vi "PDF_Interface_PDF Protokoll EPA1065_305 ARN.vi"(7 "ResultPictures":T1, 8 "error in (no error)":errorcluster caption="Fehler (Eingang, kein Fehler)", 9 "SVGraph Referenz":refnum<vi>, 10 "Save PDF File Path":path, 11 "Tabelle":string[][](table)) -> (0 "error out":errorcluster caption="Fehler (Ausgang)")   [LabVIEW 2020, in "EPA 1065.lvlib" / "ARN Test 1065-305.lvlib"]
uses:
  ARN Test 1065-305.lvlib
  T90 1065-308/Ergebnis.ctl
  PDF_Interface/PDF Interface Helper/PDFResultPictures.ctl
  Sprachverwaltung/FGV Aktion Tabelle zerlegen.ctl
  Seiten/FT-IR/FGV FT-IR Gasliste Aktionen.ctl
  Seiten/FT-IR/FGV FT-IR Aktionen.ctl
  Aktion FGV ARN Daten.ctl
  Seiten/System Einstellungen V2/Aktioen FGV System Konstanten.ctl
  PDF_Interface/PDF Protokoll Standard Kopf Optionen.ctl
  Visualisierungs Elemente/Auswahlfeld.ctl
  PDF_Interface/PDF Protokoll Standard Kopf Gasflasche Auswahl.ctl
  Aktion FGV Protokoll.ctl
  PDF_Interface/PDF Interface Helper/PDFGraph.ctl
  <vilib>/Simplicity AI/SAI_PDF_API/Classes/Context/Controls/SAI_PDF_Text Align.ctl
  PDF_Interface/PDF Interface Helper/PDFCommentPosition.ctl
  PDF_Interface/PDF Interface Helper/PDFPageBreak.ctl
  <vilib>/Simplicity AI/SAI_PDF_API/Classes/Context/Controls/SAI_PDF_PDF Details.ctl
  PDF_Interface/PDF Interface Helper/PDFContentType.ctl
  PDF_Interface/PDF Interface Helper/PDFTableContentType.ctl
  PDF_Interface/PDF Interface Helper/PDFResults.ctl
  PDF_Interface/PDF Interface Helper/PDFTablePictures.ctl
  PDF_Interface/PDF Interface Helper/PDFBemerkung.ctl
  <vilib>/Simplicity AI/SAI_PDF_API/Classes/Context/Controls/SAI_PDF_Font.ctl
  <vilib>/Simplicity AI/SAI_PDF_API/Classes/Context/Controls/SAI_PDF_Font Encoding.ctl
  Allgemein/allgemeine Sub-VIs.lvlib
  Seiten/FT-IR/FT-IR.lvlib
  Seiten/System Einstellungen V2/System Einstellungen V2.lvlib
  Sprachverwaltung/Sprachverwaltung.lvlib
  PDF_Interface/PDF Interface.lvlib
  PDF_Interface/PDF Interface Helper/PDF Interface Helper.lvlib
  <vilib>/Simplicity AI/SAI_PDF_API/Classes/Context/Context.lvclass
  Linearisierung V2/Protokoll/Protokoll.lvlib
  T90 1065-308/T90 Test 1065-308.lvlib
panel:
  out "Versa Serial number:":string caption="Serial number:"
  out "Anlage:":string caption="Measuring Device:"
  out "Einheit Noise 2":string
  out "Einheit Wiederh. 2":string
  out "Einheit Genauigkeit 2":string
  out "Einheit Noise":string
  out "Einheit Wiederh.":string
  out "Ergebnis 3":T2
  out "Ergebnis 2":T2
  out "Ergebnis 1":T2
  out "Rauschen":string
  out "Rauschen Grenze":string caption="Noise:"
  out "Wiederholgenauigkeit":string
  out "Genauigkeit":string
  out "Wiederholgenauigkeit Grenze":string caption="Repeatability:"
  out "Genauigkeit Grenze":string caption="Accuracy:"
  out "Einheit Genauigkeit":string
  out "Tabelle":string[][](table)
  out "Methode (Recipe):":string caption="Method (Recipe):"
  out "Date & Time:":string
  out "Accuracy:":string
  out "Gas Bottle Nr.:":string
  out "T90 Result":waveform(dbl)(graph) caption="T90"
  out "Ergebnis:":string caption="Result:"
  out "Konzentration:":string caption="Setpoint:"
  out "Komponente:":string caption="Component:"
  out "Bearbeiter:":string caption="Operator:"
  out "Serial number:":string
  out "Messgerät:":string caption="Analyzer:"
  # "ANR EPA § 1065.305"
  # "Limits"
  # "Results"
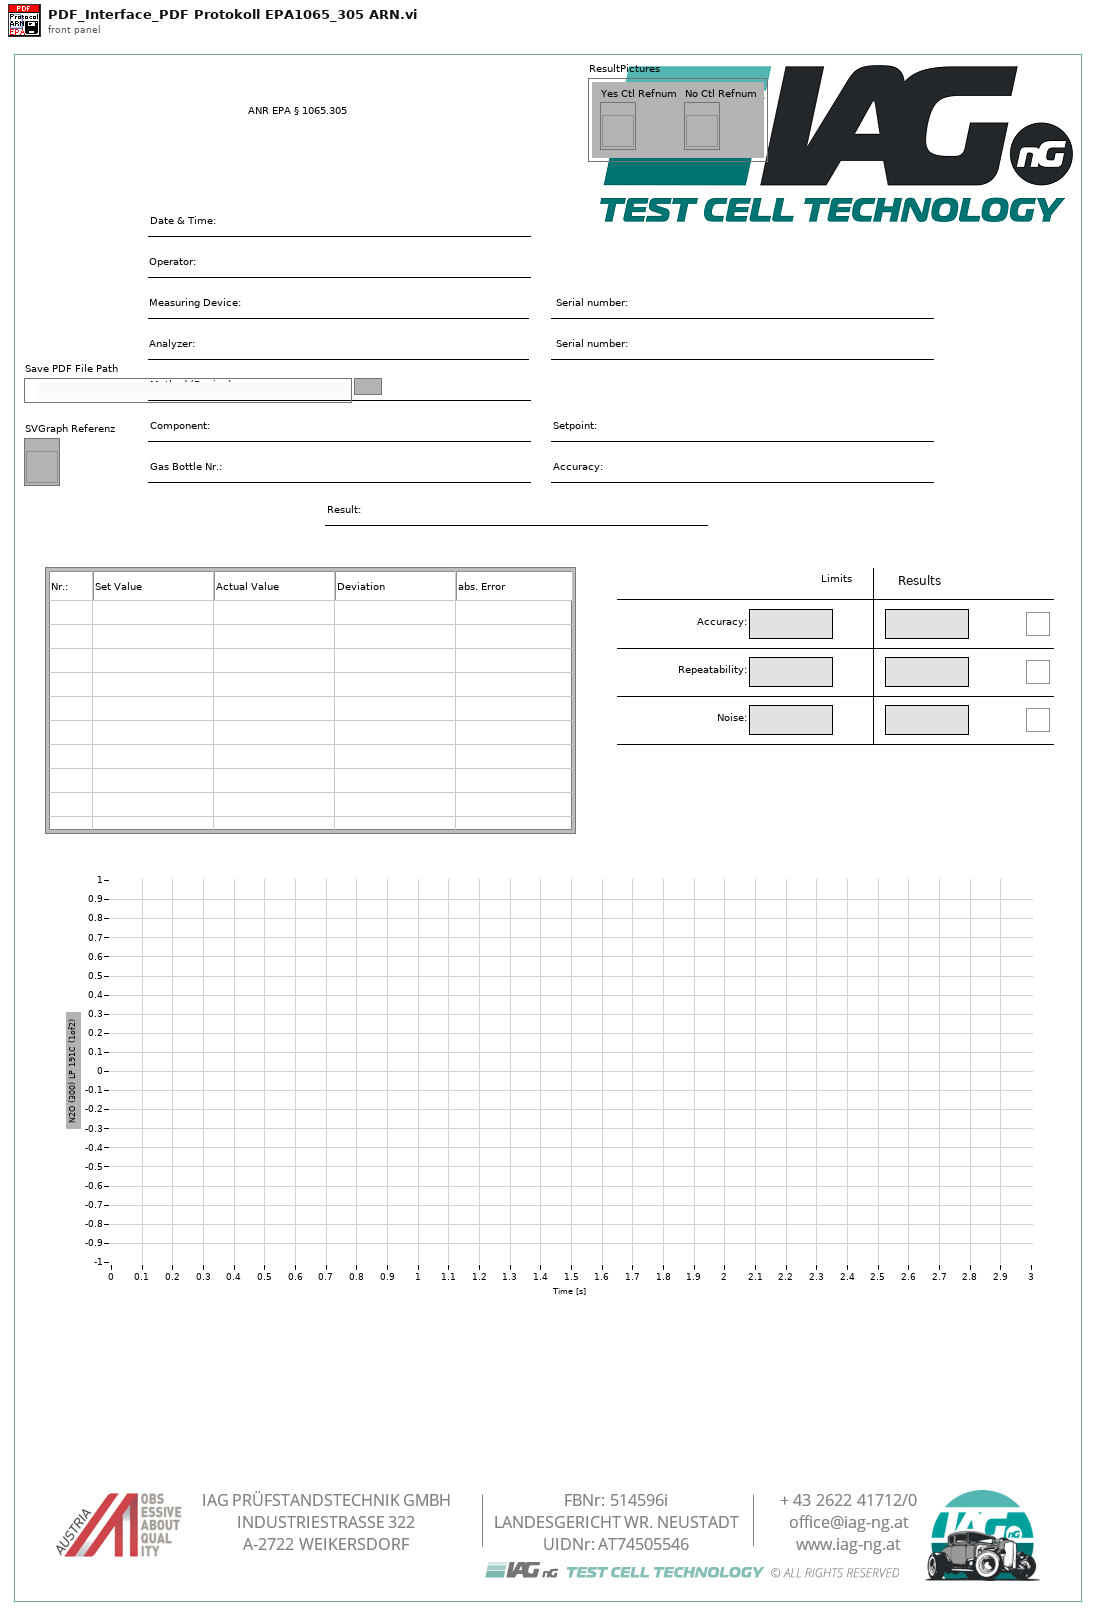
[diagram p1: front panel]
types:
  T1 = typedef "PDF Interface.lvlib/PDF Interface Helper.lvlib/PDFResultPictures.ctl" = cluster{"Yes Ctl Refnum":refnum<vi>, "No Ctl Refnum":refnum<vi>}
  T2 = typedef "EPA 1065.lvlib/T90 Test 1065-308.lvlib/Ergebnis.ctl" = bool
  T3 = typedef "Sprachverwaltung.lvlib/FGV Aktion Tabelle zerlegen.ctl" = enum16{"laden", "vereinzeln", "speichern"}
  T4 = typedef "PDF Interface.lvlib/PDF Protokoll Standard Kopf Gasflasche Auswahl.ctl" = cluster{"Gasflaschen Name":string, "Gasflaschen Nummer":string, "Gasnummer Index":i32}
  T5 = typedef "Auswahlfeld.ctl" = u16
  T6 = typedef "PDF Interface.lvlib/PDF Protokoll Standard Kopf Optionen.ctl" = cluster{"Analysator":bool, "FT-IR Rezept":bool, "Gasteiler":bool, "Gas Komponente":bool, "Gas Flasche":bool, "LIN Protokoll":bool, "Operator":bool}
  T7 = typedef "System Einstellungen V2.lvlib/Aktioen FGV System Konstanten.ctl" = enum16{"lesen", "laden", "speichern", "Sprache"}
  T8 = typedef "EPA 1065.lvlib/ARN Test 1065-305.lvlib/Aktion FGV ARN Daten.ctl" = enum16{"Lesen", "laden", "speichern", "ARN Daten", "Rohdaten", "Rohdaten löschen", "Zeitstempel", "SNR Ergebnis"}
  T9 = typedef "FT-IR.lvlib/FGV FT-IR Aktionen.ctl" = enum16{"lesen", "NOG setzen", "NOS setzen", "Initialisieren", "speichern", "ALLES setzen", "FT-IR Spektrum loggen", "Komm Stoppen", "Spektrum LogKonfig"}
  T10 = typedef "FT-IR.lvlib/FGV FT-IR Gasliste Aktionen.ctl" = enum16{"lesen", "Gasliste FT-IR", "Gasliste ausgelesen", "laden", "speichern", "löschen"}
  T11 = typedef "EPA 1065.lvlib/ARN Test 1065-305.lvlib/Aktion FGV Protokoll.ctl" = enum16{"lesen", "schreiben", "Graph"}
  T12 = typedef "PDF Interface.lvlib/PDF Interface Helper.lvlib/PDFBemerkung.ctl" = cluster{"Bemerkung Text":string, "Align (Left)":T13, "Add Line Feeds (F:No)":bool, "Font":T14}
  T13 = typedef "SAI_PDF_Toolkit.lvlib/Context.lvclass/SAI_PDF_Text Align.ctl" = i32
  T14 = typedef "SAI_PDF_Toolkit.lvlib/Context.lvclass/SAI_PDF_Font.ctl" = cluster{"Font":string, "Size":i32, "Colour":u32, "Bold":bool, "Italic":bool, "Underline":bool, "Strikethrough":bool, "Font Encoding":T15}
  T15 = typedef "SAI_PDF_Toolkit.lvlib/Context.lvclass/SAI_PDF_Font Encoding.ctl" = enum16{"Cp1252, WinANSI", "IdentityH", "IdentityV", "Cp1250", "Cp1257", "MacRoman"}
  T16 = typedef "PDF Interface.lvlib/PDF Interface Helper.lvlib/PDFContentType.ctl" = cluster{"Titel":string, "Header Table":string[][], "Table Array":T17[], "Bemerkungen":T12[]}
  T17 = typedef "PDF Interface.lvlib/PDF Interface Helper.lvlib/PDFTableContentType.ctl" = cluster{"TableHeader":string[], "Table":string[][], "Relative Column Widths (%)":sgl[], "Results":T18, "PositionBemerkung":T19, "PageBreak":T20, "TablePictures":T21, "Horizontal Align":i32}
  T18 = typedef "PDF Interface.lvlib/PDF Interface Helper.lvlib/PDFResults.ctl" = cluster{"Results":cluster{"Result Text":string, "Result":bool}[], "ResultPictures":T1, "use Pictures":bool, "Image Scale (%)":sgl, "Autoscale? (T)":bool, "Horizontal Align":i32, "Position":i32}
  T19 = typedef "PDF Interface.lvlib/PDF Interface Helper.lvlib/PDFCommentPosition.ctl" = enum16{"before", "after"}
  T20 = typedef "PDF Interface.lvlib/PDF Interface Helper.lvlib/PDFPageBreak.ctl" = enum16{"none", "before", "after", "after comment"}
  T21 = typedef "PDF Interface.lvlib/PDF Interface Helper.lvlib/PDFTablePictures.ctl" = cluster{"Ctl Refnum In":refnum<vi>[], "RowOrColumn":enum16{"Row", "Column"}, "IndexToInsert":u16, "Image Scale (%)":sgl[], "Autoscale? (T)":bool[], "Horizontal Align":i32}
  T22 = typedef "SAI_PDF_Toolkit.lvlib/Context.lvclass/SAI_PDF_PDF Details.ctl" = cluster{"Title":string, "Subject":string, "Keywords":string, "Author":string, "Creator":string}
  T23 = cluster{"Header Footer Text Cluster":cluster{"Header Text":string, "Footer Text":string, "Time":string, "Page Number":string}, "PDF Details":T22}
  T24 = typedef "EPA 1065.lvlib/ARN Test 1065-305.lvlib/Allgemeine Einstellungen.ctl" = cluster{"Bearbeiter:":string, "Analysator":T25, "Komponente:":u16, "Gasflaschen Nr.:":string, "Accuracy":dbl, "Sollwert":dbl, "Modus":T26, "Pfad:":path, "Textname:":string, "CG Aufschaltzeit:":dbl, "Einheit":string, "N2 Aufschaltzeit:":dbl, "Gasflasche":T27, "Konfig Gasflasche":T28}
  T25 = typedef "System Einstellungen V2.lvlib/Analysatoren.ctl" = string
  T26 = typedef "EPA 1065.lvlib/T90 Test 1065-308.lvlib/Modus.ctl" = u16
  T27 = typedef "System Einstellungen V2.lvlib/Gasflasche Auswahl.ctl" = u16
  T28 = typedef "System Einstellungen V2.lvlib/Konfig Gasflasche.ctl" = bool
  T29 = cluster{"Modell":string, "ProjektNummer":string, "Software Version":string, "Seriennummer":string}
  T30 = typedef "String - Ausgabefeld.ctl" = string
  T31 = cluster{"Header Size":i32, "Column Ratio left":sgl[]}
  T32 = typedef "PDF Interface.lvlib/PDF Interface Helper.lvlib/PDFGraph.ctl" = cluster{"GraphCtl Refnum":refnum<vi>, "Wrap Text (F:No)":bool, "Hide Grid (F:No)":bool, "Scale (100%)":sgl, "Align (Left)":T13, "PositionBemerkung":T19, "PageBreak":T20}
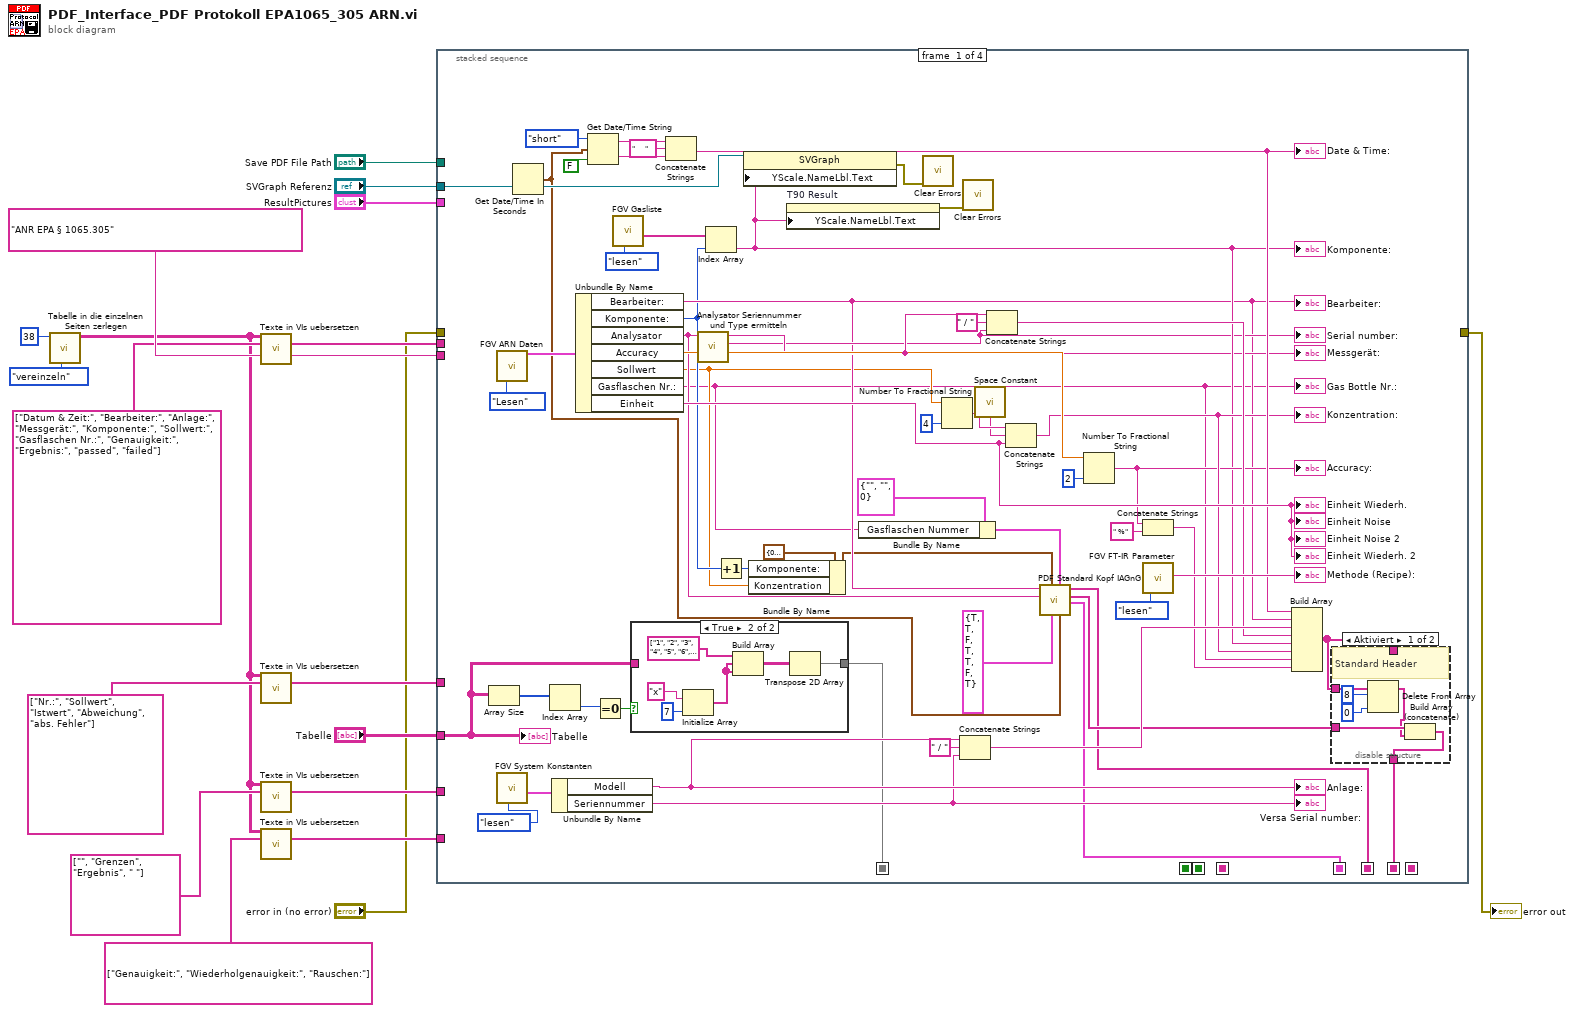
[diagram p0: block diagram]
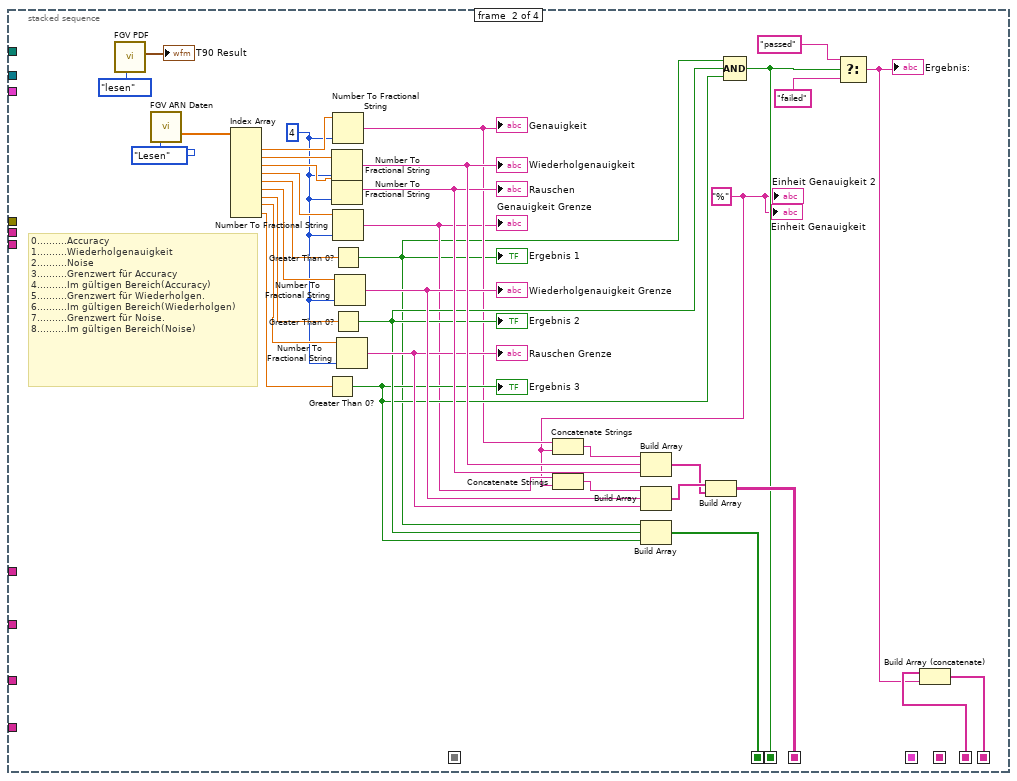
[diagram p4: hidden frame]
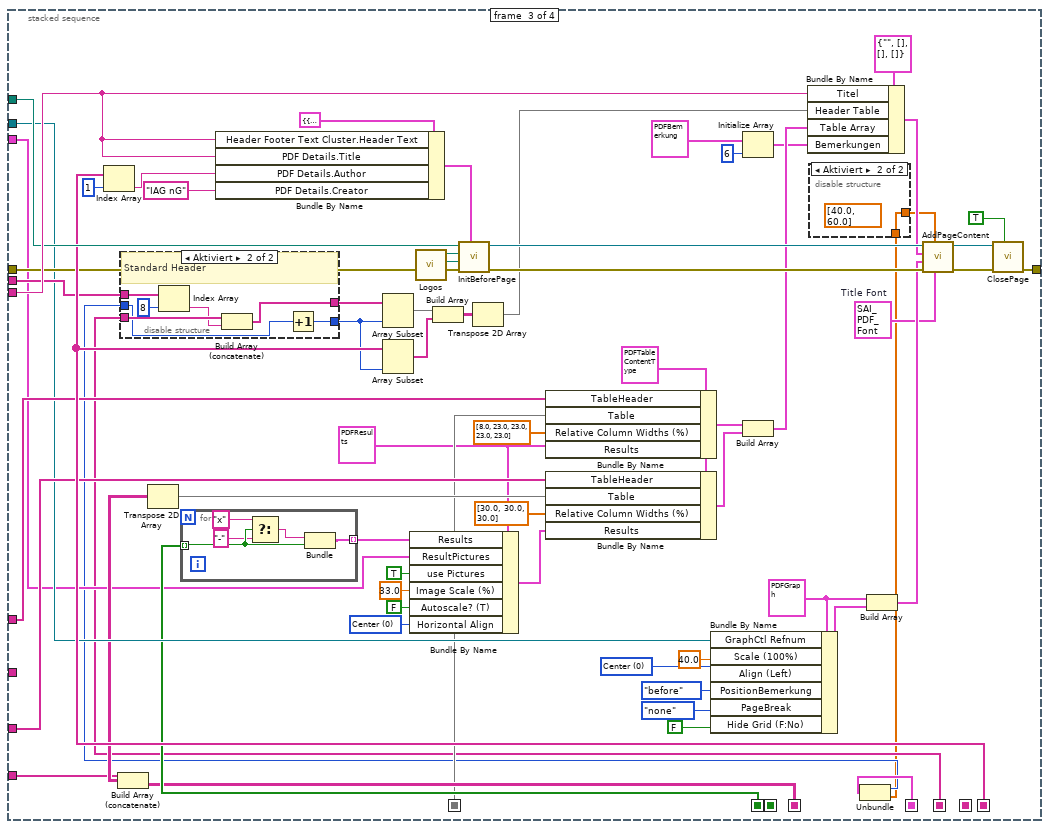
[diagram p5: hidden frame]
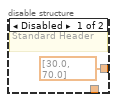
[diagram p6: hidden frame]
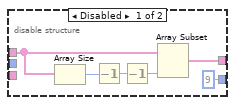
[diagram p7: hidden frame]
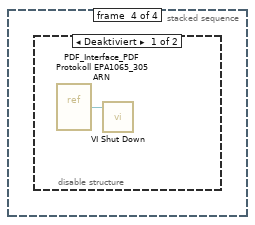
[diagram p8: hidden frame]
diagram:
  n1 = call "Tabelle in die einzelnen Seiten zerlegen.vi"("Aktion"=FGV_Aktion_Tabelle_zerlegen."vereinzeln", "Index (Seite)"=38) -> ("Sprachliste"=w8:string[][])  [unwired: 7 in, 2 out]
  n2 = call "Texte in VIs uebersetzen.vi"("Sprachliste"=w8, "String-Array zum Übersetzen"=string[] ["Datum & Zeit:", "Bearbeiter:", "Anlage:", "Messgerät:", "Komponente:", "Sollwert:", "Gasflaschen Nr.:", "Genauigkeit:", "Ergebnis:", "passed", "failed"], "String zum Übersetzen"="ANR EPA § 1065.305") -> ("String-Array zum Übersetzen"=w14:string[], "String zum Übersetzen"=w13:string)  [unwired: 8 in, 3 out]
  n3 = call "Texte in VIs uebersetzen.vi"("Sprachliste"=w8, "String-Array zum Übersetzen"=string[] ["Nr.:", "Sollwert", "Istwert", "Abweichung", "abs. Fehler"]) -> ("String-Array zum Übersetzen"=w11:string[])  [unwired: 9 in, 4 out]
  n4 = call "Texte in VIs uebersetzen.vi"("Sprachliste"=w8, "String-Array zum Übersetzen"=string[] ["", "Grenzen", "Ergebnis", " "]) -> ("String-Array zum Übersetzen"=w9:string[])  [unwired: 9 in, 4 out]
  n5 = call "Texte in VIs uebersetzen.vi"("Sprachliste"=w8, "String-Array zum Übersetzen"=string[] ["Genauigkeit:", "Wiederholgenauigkeit:", "Rauschen:"]) -> ("String-Array zum Übersetzen"=w6:string[])  [unwired: 9 in, 4 out]
  n6 = stacked-sequence {
    seq-local: [w26 _ _ _] -> [_ w111 _ _]
    seq-local: [_ w109 _ _] -> [_ _ w156 _]
    seq-local: [_ w100 _ _] -> [_ _ w148 _]
    seq-local: [_ w99 _ _] -> [_ _ w149 _]
    seq-local: [w40 _ _ _] -> [_ _ w147 _]
    seq-local: [_ w98 _ _] -> [_ _ _ _]
    seq-local: [w23 _ _ _] -> [_ _ w132 _]
    seq-local: [w22 _ _ _] -> [_ _ w130 _]
    tunnel: "Tabelle" -> [w39 _ _ _]
    tunnel: w14 -> [_ _ w153 _]
    tunnel: w13 -> [_ _ w158 _]
    tunnel: w11 -> [_ _ w152 _]
    tunnel: w9 -> [_ _ w151 _]
    tunnel: w6 -> [_ _ w145 _]
    tunnel: "Save PDF File Path" -> [_ _ w157 _]
    tunnel: "SVGraph Referenz" -> [w46 _ w150 _]
    tunnel: "error in (no error)" -> [_ _ w155 _]
    tunnel: [_ _ w154 _] -> w2
    tunnel: "ResultPictures" -> [_ _ w136 _]
    frame #0 {
      n7 = Array Size(array=w39) -> (size(s)=w43:i32[])
      n8 = call "FGV ARN Daten.vi"("Aktion"=Aktion_FGV_ARN_Daten."Lesen") -> ("ARN Konfig Daten"=w61:T24)  [unwired: 9 in, 5 out]
      n9 = call "FGV System Konstanten.vi"("Aktionen"=Aktioen_FGV_System_Konstanten."lesen") -> ("Cluster out"=w57:T29)  [unwired: 6 in, 4 out]
      n10 = Get Date/Time In Seconds() -> (seconds since 1Jan1904=w20:timestamp)
      n11 = Index Array(array=w43) -> (element=w42:i32)  [unwired: 1 in]
      n12 = Unbundle By Name(w57) -> ("Modell"=w54:string, "Seriennummer"=w53:string)
      "Versa Serial number:" <- w53
      "Anlage:" <- w54
      n13 = Unbundle By Name(w61) -> ("Bearbeiter:"=w35:string, "Komponente:"=w31:u16, "Analysator"=w34:T25, "Accuracy"=w68:dbl, "Sollwert"=w30:dbl, "Gasflaschen Nr.:"=w27:string, "Einheit"=w60:string)
      "Gas Bottle Nr.:" <- w27
      "Bearbeiter:" <- w35
      "Einheit Wiederh. 2" <- w60
      "Einheit Noise 2" <- w60
      "Einheit Noise" <- w60
      "Einheit Wiederh." <- w60
      n14 = Get Date/Time String(date format (0)=enum16{"short", "long", "abbreviated"}."short" ("Datumsformat (0)"), seconds (now)=w20, want seconds? (F)=FALSE ("Angabe von Sekunden? (F)")) -> (date string=w77:string, time string=w76:string)
      n15 = Equal To 0?(x=w42) -> (x = 0?=w41:bool)
      n16 = call "FGV Gasliste.vi"("Aktionen"=FGV_FT-IR_Gasliste_Aktionen."lesen") -> ("Aktuelle Gasliste gesamt"=w71:T30[])  [unwired: 8 in, 2 out]
      n17 = case shown="True" w41 {
        tunnel: [w85 w86] -> w40
        tunnel: w39 -> [w85 _]
        frame False {
        }
        frame True {
          n18 = Initialize Array("x", 7 ("Dimensionsgröße")) -> (w88:string[])
          n19 = Build Array(string[] ["1", "2", "3", "4", "5", "6", "7"], w88, w88) -> (w87:string[][])
          n20 = Transpose 2D Array(2D array=w87) -> (transposed array=w86:string[][])
        }
      }
      n21 = Concatenate Strings(w77, "     " ("String"), w76) -> (w58:string)
      "Date & Time:" <- w58
      n22 = call "Analysator Seriennummer und Type ermitteln.vi"("Analysator"=w34) -> ("Type"=w37:string, "Name für Protokoll"=w38:string)  [unwired: 8 in, 1 out]
      "Messgerät:" <- w38
      "Serial number:" <- w37
      n23 = Index Array(array=w71, index=w31) -> (element=w44:T30)
      "Komponente:" <- w44
      n24 = Increment(x=w31) -> (x+1=w21:u16)
      n25 = property class="SVGraph"(reference=w46, "YScale.NameLbl.Text"=w44) -> (error out=w45:errorcluster)  [unwired: 1 in, 1 out]
      n26 = Bundle By Name(cluster=cluster{"Komponente:":T5, "Konzentration":dbl} {"Komponente:"=0, "Konzentration"=0.0} ("Gas Komponente"), "Komponente:"=w21, "Konzentration"=w30) -> (w32:cluster{"Komponente:":T5, "Konzentration":dbl})
      n27 = property on="T90 Result" class="SVGraph (strikt)"("YScale.NameLbl.Text"=w44) -> (error out=w65:errorcluster)  [unwired: 2 in, 1 out]
      n28 = Bundle By Name(cluster=T4 {"Gasflaschen Name"="", "Gasflaschen Nummer"="", "Gasnummer Index"=0} ("Gaschflasche Cluster"), "Gasflaschen Nummer"=w27) -> (w28:T4)
      n29 = call <vilib>:"Clear Errors.vi"("error in (no error)"=w45) -> ()  [unwired: 5 in, 2 out]
      n30 = Number To Fractional String(number=w30, precision (6)=i16 4 ("Genauigkeit (6)")) -> (F-format string=w64:string)  [unwired: 2 in]
      n31 = Concatenate Strings(w54, " / " ("String"), w53) -> (w52:string)
      n32 = call <vilib>:"Clear Errors.vi"("error in (no error)"=w65) -> ()  [unwired: 5 in, 2 out]
      n33 = call <vilib>:"Space Constant.vi"() -> ("String"=w63:string)
      n34 = Concatenate Strings(w38, " / " ("String"), w37) -> (w51:string)
      n35 = Concatenate Strings(w64, w63, w60) -> (w50:string)
      "Konzentration:" <- w50
      n36 = call "PDF Standard Kopf IAGnG.vi"("Zeitstempel"=w20, "Gaschflasche Cluster"=w28, "Oprtionen Cluster"=T6 {"Analysator"=TRUE, "FT-IR Rezept"=TRUE, "Gasteiler"=FALSE, "Gas Komponente"=TRUE, "Gas Flasche"=TRUE, "LIN Protokoll"=FALSE, "Operator"=TRUE}, "Gas Komponente"=w32, "Analysator"=w34, "Bearbeiter/in"=w35) -> ("Size Cluster"=w22:T31, "Header Values"=w24:T30[], "Header Labels"=w23:string[])  [unwired: 2 in, 1 out]
      n37 = Number To Fractional String(number=w68, precision (6)=i16 2 ("Genauigkeit (6)")) -> (F-format string=w49:string)  [unwired: 2 in]
      "Accuracy:" <- w49
      n38 = Concatenate Strings(w49, " %" ("String")) -> (w47:string)
      n39 = call "FGV FT-IR Parameter.vi"("Aktion"=FGV_FT-IR_Aktionen."lesen") -> ("Current Recipe"=→"Methode (Recipe):":string)  [unwired: 11 in, 7 out]
      n40 = Build Array(w58, w35, w52, w51, w44, w50, w27, w47) -> (w25:T30[])
      n41 = disable-structure shown="Aktiviert" {
        disable-tunnel: w25 -> [w83 _]
        disable-tunnel: [w78 w84] -> w26
        disable-tunnel: w25 -> [_ w84]
        disable-tunnel: w24 -> [w80 _]
        frame Enabled {
          # "Standard Header"
          n42 = Delete From Array(array=w83, length=8 ("Länge"), index=0 ("Index")) -> (array with subset deleted=w79:T30[])  [unwired: 1 out]
          n43 = Build Array (concatenate)(w80, w79) -> (w78:T30[])
        }
        frame Disabled {
        }
      }
      "Tabelle" <- w39
    }
    frame #1 {
      w93 = "%" ("Einheit Genauigkeit 2")
      w113 = i16 4 ("Genauigkeit (6)")
      # "0..........Accuracy\n1..........Wiederholgenauigkeit\n2..........Noise\n3..........Grenzwert für Accuracy\n4..........Im gültigen Bereich(Accuracy)\n5..........Grenzwert für Wiederholgen.\n6..........Im gültigen Bereich(Wiederholgen)\n7..........Grenzwert für Noise.\n8..........Im gültigen Bereich(Noise)"
      n44 = call "FGV PDF.vi"("Aktion"=Aktion_FGV_Protokoll."lesen") -> ("Graph"=→"T90 Result":waveform(dbl))  [unwired: 9 in, 1 out]
      n45 = call "FGV ARN Daten.vi"("Aktion"=Aktion_FGV_ARN_Daten."Lesen") -> ("SNR Ergebnis"=w114:sgl[])  [unwired: 9 in, 5 out]
      n46 = Index Array(array=w114) -> (element #1=w115:sgl, element #2=w116:sgl, element #3=w117:sgl, element #4=w118:sgl, element #5=w119:sgl, element #6=w120:sgl, element #7=w121:sgl, element #8=w122:sgl, element #9=w123:sgl)  [unwired: 9 in]
      n47 = Greater Than 0?(x=w123) -> (x > 0?=w103:bool)
      "Ergebnis 3" <- w103
      n48 = Number To Fractional String(number=w116, precision (6)=w113) -> (F-format string=w108:string)  [unwired: 2 in]
      "Wiederholgenauigkeit" <- w108
      n49 = Number To Fractional String(number=w117, precision (6)=w113) -> (F-format string=w107:string)  [unwired: 2 in]
      "Rauschen" <- w107
      n50 = Number To Fractional String(number=w115, precision (6)=w113) -> (F-format string=w97:string)  [unwired: 2 in]
      "Genauigkeit" <- w97
      n51 = Number To Fractional String(number=w118, precision (6)=w113) -> (F-format string=w95:string)  [unwired: 2 in]
      "Genauigkeit Grenze" <- w95
      n52 = Greater Than 0?(x=w119) -> (x > 0?=w92:bool)
      "Ergebnis 1" <- w92
      n53 = Greater Than 0?(x=w121) -> (x > 0?=w104:bool)
      "Ergebnis 2" <- w104
      n54 = Number To Fractional String(number=w120, precision (6)=w113) -> (F-format string=w106:string)  [unwired: 2 in]
      "Wiederholgenauigkeit Grenze" <- w106
      n55 = Number To Fractional String(number=w122, precision (6)=w113) -> (F-format string=w105:string)  [unwired: 2 in]
      "Rauschen Grenze" <- w105
      n56 = Concatenate Strings(w97, w93) -> (w96:string)
      n57 = Concatenate Strings(w95, w93) -> (w94:string)
      n58 = Build Array(w96, w108, w107) -> (w101:string[])
      n59 = Build Array(w94, w106, w105) -> (w102:string[])
      n60 = Build Array(w92, w104, w103) -> (w99:bool[])
      n61 = Build Array(w102, w101) -> (w100:string[][])
      n62 = Compound Arithmetic op=AND ("Mehrfacharithmetik")(w92, w104, w103) -> (w98:bool)
      n63 = Select(t="passed", s=w98, f="failed") -> (s? t:f=w110:string)
      "Ergebnis:" <- w110
      n64 = Build Array (concatenate)(w111, w110) -> (w109:T30[])
      "Einheit Genauigkeit 2" <- w93
      "Einheit Genauigkeit" <- w93
    }
    frame #2 {
      w135 = T13 0 items=["Center", "Justified", "Justified All", "Left", "Right"] ("Align (Left)")
      w142 = T18 {"Results"=[], "ResultPictures"={"Yes Ctl Refnum"=refnum, "No Ctl Refnum"=refnum}, "use Pictures"=FALSE, "Image Scale (%)"=100.0, "Autoscale? (T)"=TRUE, "Horizontal Align"=3, "Position"=0} ("Results")
      w144 = T17 {"TableHeader"=[], "Table"=[], "Relative Column Widths (%)"=[], "Results"={"Results"=[], "ResultPictures"={"Yes Ctl Refnum"=refnum, "No Ctl Refnum"=refnum}, "use Pictures"=FALSE, "Image Scale (%)"=0.0, "Autoscale? (T)"=FALSE, "Horizontal Align"=0, "Position"=0}, "PositionBemerkung"=enum."before", "PageBreak"=enum."none", "TablePictures"={"Ctl Refnum In"=[], "RowOrColumn"=enum."Row", "IndexToInsert"=0, "Image Scale (%)"=[], "Autoscale? (T)"=[], "Horizontal Align"=0}, "Horizontal Align"=0} ("Table Content")
      w165 = T14 {"Font"="Arial", "Size"=26, "Colour"=0, "Bold"=TRUE, "Italic"=FALSE, "Underline"=TRUE, "Strikethrough"=FALSE, "Font Encoding"=enum."Cp1252, WinANSI"}  # Title Font
      w169 = T13 0 items=["Center", "Justified", "Justified All", "Left", "Right"] ("Align (Left)")
      w162 = T32 {"GraphCtl Refnum"=refnum, "Wrap Text (F:No)"=FALSE, "Hide Grid (F:No)"=FALSE, "Scale (100%)"=100.0, "Align (Left)"=0, "PositionBemerkung"=enum."before", "PageBreak"=enum."after comment"} ("Graph")
      n65 = Index Array(array=w156, index=1 ("Index")) -> (element=w159:T30)
      n66 = Build Array (concatenate)(w145, w148) -> (w146:string[][])
      n67 = Transpose 2D Array(2D array=w146) -> (transposed array=w161:string[][])
      n68 = for {
        tunnel: w149 -> [w212] mode=indexing
        tunnel: [w213] -> w141 mode=indexing
        n69 = Select(t="x", s=w212, f="-") -> (s? t:f=w209:string)
        n70 = Bundle(w209, w212) -> (w213:cluster{string, bool})  [unwired: 1 in]
      }
      n71 = Bundle By Name(cluster=T23 {"Header Footer Text Cluster"={"Header Text"="Protokoll XYZ", "Footer Text"="IAG nG", "Time"="<TIMESTAMP yyyy-MM-dd>", "Page Number"="Page <P> of <PT>"}, "PDF Details"={"Title"="Test PDF", "Subject"="Versa Tabasco", "Keywords"="", "Author"="RIW", "Creator"="IAG"}} ("Info"), "Header Footer Text Cluster.Header Text"=w158, "PDF Details.Title"=w158, "PDF Details.Author"=w159, "PDF Details.Creator"="IAG nG") -> (w184:T23)
      n72 = Bundle By Name(cluster=w142, "Results"=w141, "ResultPictures"=w136, "use Pictures"=TRUE, "Image Scale (%)"=sgl 33.0, "Autoscale? (T)"=FALSE, "Horizontal Align"=w135) -> (w143:T18)
      n73 = call "Logos.vi"() -> ("Footer Image File Path"=w192:path, "Header Image File Path"=w193:path)  [unwired: 8 in, 2 out]
      n74 = call "InitBeforePage.vi"("Info"=w184, "Fehler (Eingang, kein Fehler)"=w155, "Footer Image File Path"=w192, "Header Image File Path"=w193, "Path (Dialog if Empty)"=w157) -> ("Fehler (Ausgang)"=w191:errorcluster, "Context (Ausgang)"=w190:refnum<class "Context.lvclass">)  [unwired: 5 in]
      n75 = Bundle By Name(cluster=w144, "TableHeader"=w152, "Table"=w147, "Relative Column Widths (%)"=sgl[] [8.0, 23.0, 23.0, 23.0, 23.0], "Results"=w142) -> (w177:T17)
      n76 = Bundle By Name(cluster=w144, "TableHeader"=w151, "Table"=w161, "Relative Column Widths (%)"=sgl[] [30.0, 30.0, 30.0], "Results"=w143) -> (w164:T17)
      n77 = Bundle By Name(cluster=w162, "GraphCtl Refnum"=w150, "Scale (100%)"=sgl 40.0, "Align (Left)"=w169, "PositionBemerkung"=PDFCommentPosition."before", "PageBreak"=PDFPageBreak."none", "Hide Grid (F:No)"=FALSE) -> (w173:T32)
      n78 = Initialize Array(T12 {"Bemerkung Text"="", "Align (Left)"=0, "Add Line Feeds (F:No)"=FALSE, "Font"={"Font"="Arial", "Size"=10, "Colour"=0, "Bold"=FALSE, "Italic"=FALSE, "Underline"=FALSE, "Strikethrough"=FALSE, "Font Encoding"=enum."Cp1252, WinANSI"}} ("Bemerkung"), 6 ("Dimensionsgröße")) -> (w134:T12[])
      n79 = Build Array(w177, w164) -> (w140:T17[])
      n80 = Unbundle(w130) -> ("Header Size"=w129:i32, "Column Ratio left"=w128:sgl[])
      n81 = disable-structure shown="Aktiviert" {
        disable-tunnel: [w198 w207] -> w179
        disable-tunnel: w153 -> [w197 w206]
        disable-tunnel: w132 -> [_ w208]
        disable-tunnel: w129 -> [_ w203]
        disable-tunnel: [9 ("Länge") w202] -> w131
        frame Disabled {
          n82 = Array Size(array=w197) -> (size(s)=w201:i32)
          n83 = Decrement(x=w201) -> (x-1=w200:i32)
          n84 = Decrement(x=w200) -> (x-1=w199:i32)
          n85 = Array Subset(array=w197, length=w199) -> (w198:string[])  [unwired: 1 in]
        }
        frame Enabled {
          # "Standard Header"
          n86 = Index Array(array=w206, index=8 ("Index")) -> (element=w204:string)
          n87 = Build Array (concatenate)(w208, w204) -> (w207:string[])
          n88 = Increment(x=w203) -> (x+1=w202:i32)
        }
      }
      n89 = Array Subset(array=w179, length=w131) -> (w182:string[])  [unwired: 1 in]
      n90 = Array Subset(array=w156, length=w131) -> (w181:T30[])  [unwired: 1 in]
      n91 = Build Array(w182, w181) -> (w180:T30[][])
      n92 = Transpose 2D Array(2D array=w180) -> (transposed array=w174:T30[][])
      n93 = Bundle By Name(cluster=T16 {"Titel"="", "Header Table"=[], "Table Array"=[], "Bemerkungen"=[]} ("Content"), "Titel"=w158, "Header Table"=w174, "Table Array"=w140, "Bemerkungen"=w134) -> (w176:T16)
      n94 = disable-structure shown="Aktiviert" {
        disable-tunnel: [sgl[] [30.0, 70.0] ("Column Ratio left") w195] -> w175
        disable-tunnel: w128 -> [_ w195]
        frame Disabled {
          # "Standard Header"
        }
        frame Enabled {
          (unwired) sgl[] [40.0, 60.0] ("Column Ratio left")
        }
      }
      n95 = Build Array(w162, w173) -> (w167:T32[])
      n96 = call "AddPageContent.vi"("Title Font"=w165, "Column Ratio left"=w175, "error in"=w191, "Graph Array"=w167, "Content"=w176, "Context (Eingang)"=w190) -> ("error out"=w189:errorcluster, "Context (Ausgang)"=w188:refnum<class "Context.lvclass">)  [unwired: 4 in]
      n97 = call "ClosePage.vi"("popup viewer"=TRUE, "Fehler (Eingang, kein Fehler)"=w189, "Context (Eingang)"=w188) -> ("Fehler (Ausgang)"=w154:errorcluster)  [unwired: 8 in]
    }
    frame #3 {
      n98 = disable-structure shown="Deaktiviert" {
        frame Disabled {
          n99 = vi-ref "PDF_Interface_PDF Protokoll EPA1065_305 ARN.vi"() -> (w214:refnum<vi>)
          n100 = call "VI Shut Down.vi"("VI Referenz"=w214) -> ()  [unwired: 11 in]
        }
        frame Enabled {
        }
      }
    }
  }
  "error out" <- w2
